vi "hw7p5_hickey.vi"() -> ()   [LabVIEW 2014]
uses:
  <vilib>/MakerHub/LINX/Private/Type Defs/User Platform.ctl
  <vilib>/MakerHub/LINX/Private/Type Defs/Interface.ctl
  <vilib>/MakerHub/LINX/Public/Peripherals/Analog/Analog Read 1 Chan.vi
  <vilib>/MakerHub/LINX/Public/Peripherals/Digital/Digital Write 1 Chan.vi
  <vilib>/MakerHub/LINX/LMH-LINX.lvlib
panel:
  out "Error Out 8":errorcluster
  out "Error Out 7":errorcluster
  out "Error Out 6":errorcluster
  in  "Temp 4":dbl
  in  "DO Channel 3":u8
  out "Error Out 5":errorcluster
  in  "Temp 3":dbl
  in  "Temp 2":dbl
  out "Error Out 4":errorcluster
  in  "DO Channel 2":u8
  out "Error Out 3":errorcluster
  in  "stop":bool
  out "Error Out 2":errorcluster
  out "Error Out":errorcluster
  in  "Temp1":dbl
  out "AI Value":dbl
  in  "DO Channel":u8
  in  "Analog Channel":u8
  in  "Serial Port":refnum<visa-resource-name>="N/A"
  in  "Interface":T1
  in  "Platform":T2
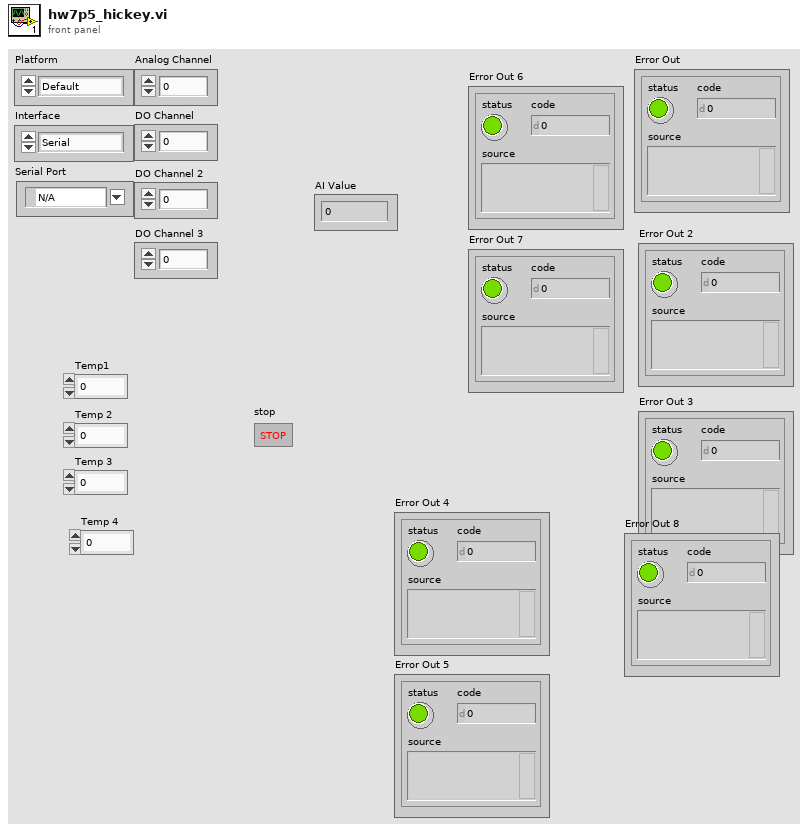
[diagram p1: front panel]
types:
  T1 = typedef "LMH-LINX.lvlib/Interface.ctl" = enum16{"Serial", "TCP"}
  T2 = typedef "LMH-LINX.lvlib/User Platform.ctl" = enum16{"Default", "LINX", "myRIO"}
  T3 = typedef "LMH-LINX.lvlib/LINX Ref.ctl" = cluster{"Platform":T4, "Interface":T1, "LINX Device Config":T5}
  T4 = typedef "LMH-LINX.lvlib/Platform.ctl" = enum16{"LINX", "myRIO"}
  T5 = typedef "LMH-LINX.lvlib/Device.lvlib/LINX Device Config.ctl" = cluster{"Interface":T1, "COM Port":refnum<visa-resource-name>, "TCP Configuration":T6, "Device Family":u8, "Device ID":u8, "Device Name":string, "TCP Ref":refnum<k5>, "Channels":T7}
  T6 = typedef "LMH-LINX.lvlib/Device.lvlib/TCP Config.ctl" = cluster{"IP Address":string, "Port":u16}
  T7 = typedef "LMH-LINX.lvlib/Channels.ctl" = cluster{"DI":u8[], "DO":u8[], "AI":u8[], "AO":u8[], "PWM":u8[], "QE":u8[], "UART":u8[], "I2C 2":u8[], "SPI":u8[], "CAN":u8[], "Servo":u8[], "AI Ref (V)":dbl, "AO Ref (V)":dbl, "AO Resolution (Bits)":u8}
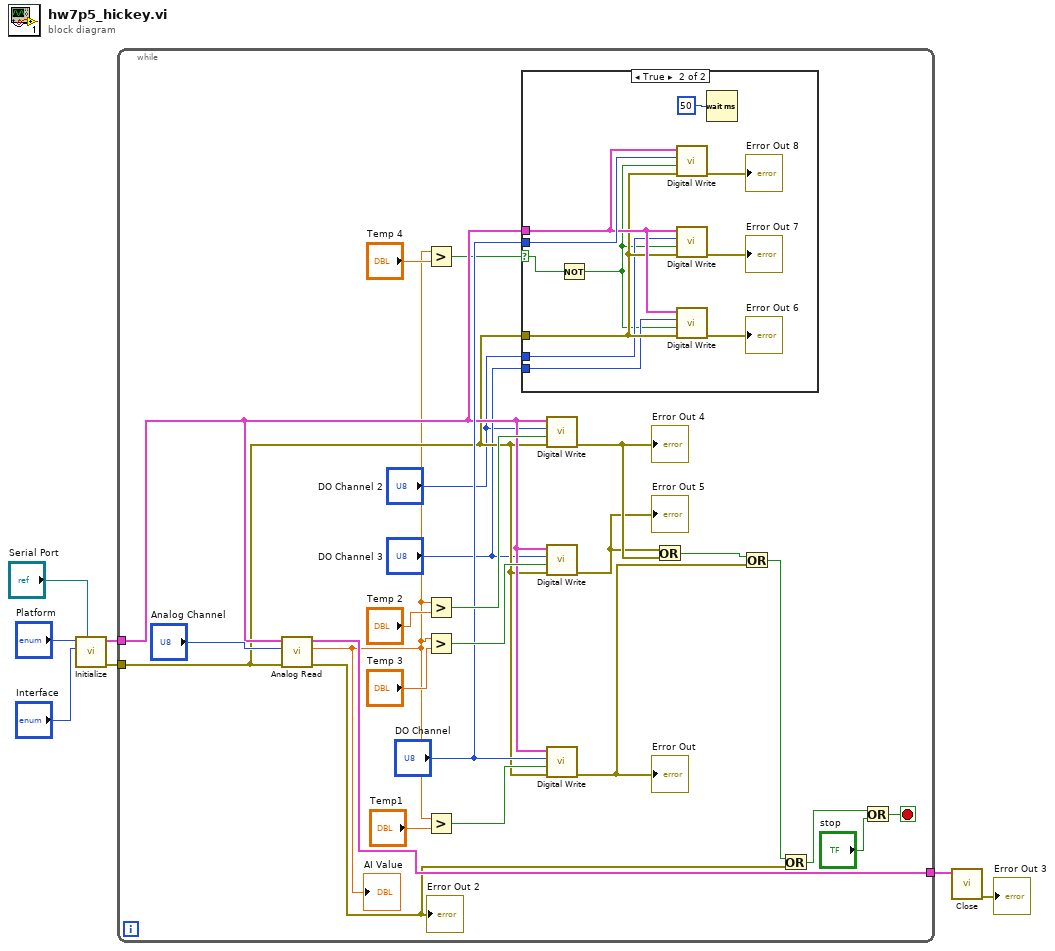
[diagram p0: block diagram]
diagram:
  n1 = call <vilib>:"Initialize.vi"("Serial Port"="Serial Port", "Interface"="Interface", "Platform"="Platform") -> ("Error Out"=w2:errorcluster, "LINX Ref"=w6:T3)  [unwired: 6 in, 1 out]
  n2 = while {
    tunnel: [w32] -> w7
    tunnel: w6 -> [w15]
    tunnel: w2 -> [w14]
    stop <- w26 stop-if-true
    n3 = call-poly <vilib>:"Analog Read.vi"("Error In"=w14, "Analog Channel"="Analog Channel", "LINX Resource"=w15) -> ("Error Out"=w29:errorcluster, "AI Value"=w8:dbl, "LINX Resource"=w32:T3)  [unwired: 5 in, 1 out]
    "AI Value" <- w8
    "Error Out 2" <- w29
    n4 = Greater?(x=w8, y="Temp 4") -> (0:w11:bool)
    n5 = Greater?(x=w8, y="Temp 2") -> (0:w25:bool)
    n6 = Greater?(x=w8, y="Temp 3") -> (0:w19:bool)
    n7 = Greater?(x=w8, y="Temp1") -> (0:w30:bool)
    n8 = case shown="True" w11 {
      selector: w11 -> [_ w34]
      tunnel: "DO Channel" -> [_ w39]
      tunnel: w15 -> [_ w38]
      tunnel: w14 -> [_ w37]
      tunnel: "DO Channel 3" -> [_ w36]
      tunnel: "DO Channel 2" -> [_ w35]
      frame False {
      }
      frame True {
        n9 = Not(x=w34) -> (.not. x?=w33:bool)
        n10 = call-poly <vilib>:"Digital Write.vi"("Error In"=w37, "Output Value"=w33, "DO Channel"=w39, "LINX Resource"=w38) -> ("Error Out"=→"Error Out 8":errorcluster)  [unwired: 6 in, 1 out]
        n11 = call-poly <vilib>:"Digital Write.vi"("Error In"=w37, "Output Value"=w33, "DO Channel"=w35, "LINX Resource"=w38) -> ("Error Out"=→"Error Out 7":errorcluster)  [unwired: 6 in, 1 out]
        n12 = call-poly <vilib>:"Digital Write.vi"("Error In"=w37, "Output Value"=w33, "DO Channel"=w36, "LINX Resource"=w38) -> ("Error Out"=→"Error Out 6":errorcluster)  [unwired: 6 in, 1 out]
        n13 = Wait (ms)(milliseconds to wait=u32 50) -> ()  [unwired: 1 out]
      }
    }
    n14 = call-poly <vilib>:"Digital Write.vi"("Error In"=w14, "Output Value"=w25, "DO Channel"="DO Channel 2", "LINX Resource"=w15) -> ("Error Out"=w22:errorcluster)  [unwired: 6 in, 1 out]
    "Error Out 4" <- w22
    n15 = call-poly <vilib>:"Digital Write.vi"("Error In"=w14, "Output Value"=w19, "DO Channel"="DO Channel 3", "LINX Resource"=w15) -> ("Error Out"=w20:errorcluster)  [unwired: 6 in, 1 out]
    "Error Out 5" <- w20
    n16 = call-poly <vilib>:"Digital Write.vi"("Error In"=w14, "Output Value"=w30, "DO Channel"="DO Channel", "LINX Resource"=w15) -> ("Error Out"=w24:errorcluster)  [unwired: 6 in, 1 out]
    "Error Out" <- w24
    n17 = Or(x=w20, y=w22) -> (x .or. y?=w21:bool)
    n18 = Or(x=w21, y=w24) -> (x .or. y?=w23:bool)
    n19 = Or(x=w23, y=w29) -> (x .or. y?=w28:bool)
    n20 = Or(x=w28, y="stop") -> (x .or. y?=w26:bool)
  }
  n21 = call <vilib>:"Close.vi"("LINX Resource"=w7) -> ("Error Out"=→"Error Out 3":errorcluster)  [unwired: 9 in, 1 out]
